vi "toStringArray.vi"(8 "error in (no error)":errorcluster, 11 "RampToneAmplitudeUp in":refnum<class "RampToneAmplitudeUp.lvclass">) -> (0 "error out":errorcluster, 2 "eventStringArray":string[](array[string]), 3 "RampToneAmplitudeUp out":refnum<class "RampToneAmplitudeUp.lvclass">)   [LabVIEW 2011, in "Tools.lvlib" / "Scripting.lvlib" / "RampToneAmplitudeUp.lvclass"]
uses:
  RampToneAmplitudeUp.lvclass
  RampTone/RampTone.lvclass
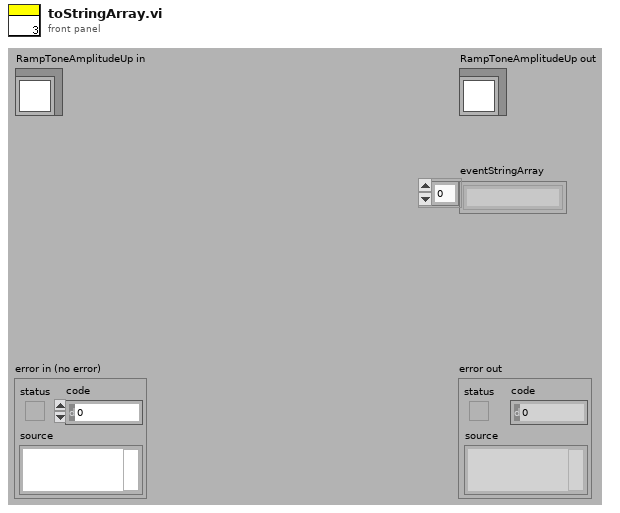
[diagram p1: front panel]
types:
  T1 = cluster{"rampTime":dbl, "timeStep":dbl, "dataValueStep":dbl}
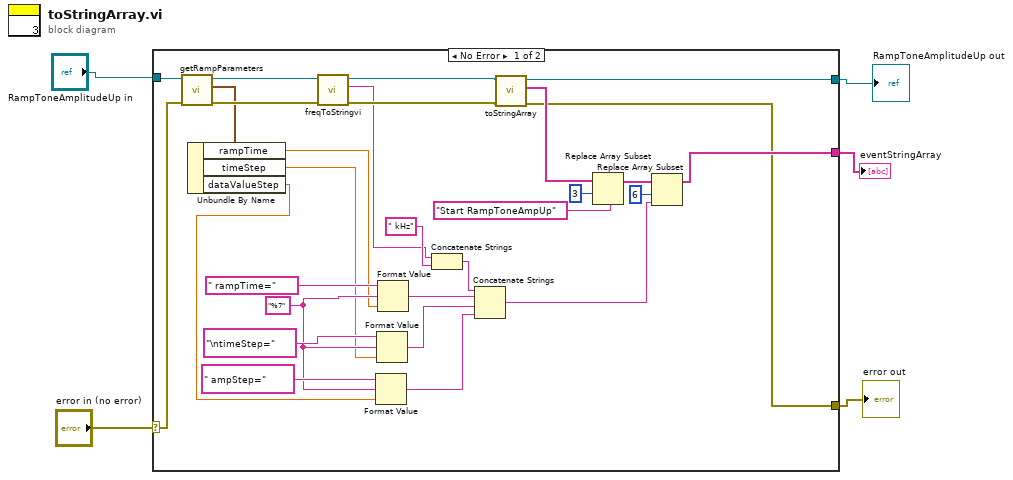
[diagram p0: block diagram]
diagram:
  n1 = case shown="No Error" "error in (no error)" {
    selector: "error in (no error)" -> [w13 w35]
    tunnel: [w16 w35] -> w1
    tunnel: [w24 _] -> w2
    tunnel: "RampToneAmplitudeUp in" -> [w14 w36]
    tunnel: [w19 w36] -> w3
    frame No Error {
      w23 = "%7"
      n2 = call "getRampParameters.vi"("error in (no error)"=w13, "RampTone in"=w14) -> ("error out"=w12:errorcluster, "RampParameters"=w11:T1, "RampTone out"=w10:refnum<class "RampToneAmplitudeUp.lvclass">)  [unwired: 7 in]
      n3 = Unbundle By Name(w11) -> ("rampTime"=w9:dbl, "timeStep"=w8:dbl, "dataValueStep"=w7:dbl)
      n4 = call-dynamic "freqToStringvi.vi"("error in (no error)"=w12, "SingleTone in"=w10) -> ("error out"=w17:errorcluster, "frequency"=w6:string, "SingleTone out"=w20:refnum<class "RampToneAmplitudeUp.lvclass">)  [unwired: 7 in]
      n5 = Format Value(string ("")=" ampStep=", format string=w23, value (0)=w7) -> (output string=w15:string)
      n6 = Format Value(string ("")="\ntimeStep=", format string=w23, value (0)=w8) -> (output string=w26:string)
      n7 = Format Value(string ("")=" rampTime=", format string=w23, value (0)=w9) -> (output string=w27:string)
      n8 = Concatenate Strings(w6, " kHz") -> (w21:string)
      n9 = Concatenate Strings(w21, w27, w26, w15) -> (w25:string)
      n10 = call-parent "toStringArray.vi"("error in (no error)"=w17, "RampTone in"=w20) -> ("error out"=w16:errorcluster, "eventStringArray"=w18:string[], "RampTone out"=w19:refnum<class "RampToneAmplitudeUp.lvclass">)  [unwired: 7 in]
      n11 = Replace Array Subset(array=w18, new element="Start RampToneAmpUp", index=3) -> (w30:string[])
      n12 = Replace Array Subset(array=w30, new element=w25, index=6) -> (w24:string[])
    }
    frame Error {
    }
  }
  "error out" <- w1
  "RampToneAmplitudeUp out" <- w3
  "eventStringArray" <- w2
